vi "GameToIAStateKeeper.vi"(8 "error in (no error)":errorcluster, 11 "Game in":refnum<class "Game.lvclass">) -> (0 "error out":errorcluster, 2 "IA State out":T1={"our_robots"=[], "enemy_robots"=[], "balls"=[], "geometry"={"line_width"=0, "field_length"=0, "field_width"=0, "boundary_width"=0, "referee_width"=0, "goal_width"=0, "goal_depth"=0, "goal_wall_width"=0, "center_circle_radius"=0, "defense_radius"=0, "defense_stretch"=0, "free_kick_from_defense_dist"=0, "penalty_spot_from_field_line_dist"=0, "penalty_line_from_spot_dist"=0}, "IA Judge"={"stage"="", "command"="", "our_goalie_id"=0.0, "enemy_goalie_id"=0.0, "command enum"=enum."Halt", "Time"=enum."Azul", "Point"={"x"=0.0, "y"=0.0}}, "Received Timestamp"=timestamp(0 s since 1904-01-01), "Events"={"Touch"=FALSE, "Ball out"=FALSE, "id touch"=0.0, "Ball out of \nVision"=FALSE, "Ball inside \nGoalie area"=FALSE, "Robot not responding"=FALSE, "Robots responding status"=[1.0, 1.0, 1.0, 1.0, 1.0, 1.0], "Enemy Ball \nPossession"=FALSE, "Pass State"=FALSE, "id end of pass"=0.0, "Kick"=FALSE, "Id ini Possession"=0.0, "Ball Possesion"=FALSE, "Id Possesion"=0.0, "Direct Kick"=FALSE, "2nd Strk Ativo"=FALSE}}, 3 "Game out":refnum<class "Game.lvclass">, 6 "Parameters.lvclass":refnum<class "Parameters.lvclass">)   [LabVIEW 2023, in "Game.lvclass"]
uses:
  Game.lvclass
  Vision_class/Old vision/SSL Detection Frame Simple Estimator Cameras VelCmd Folder/Core/AI Input.ctl
  Vision_class/Old vision/Controls/AI Robot.ctl
  Vision_class/Old vision/Controls/Functions Enum.ctl
  Controls/estimatives.ctl
  Vision_class/Old vision/Controls/AttackerStates.ctl
  Vision_class/Old vision/Controls/PathDests.ctl
  Vision_class/Old vision/Controls/PathDest.ctl
  Navigation/VSSNavigation/VSSAttackerStates.ctl
  Robot_class/robotKickToStates.ctl
  Robot_class/roles.ctl
  <vilib>/Analysis/Matrix/Datatypes/RealMatrix.ctl
  Navigation/driveMode.ctl
  Vision_class/Old vision/SSL Detection Frame Simple Estimator Cameras VelCmd Folder/Core/AI Ball.ctl
  Vision_class/Old vision/SSL Detection Frame Simple Estimator Cameras VelCmd Folder/Core/Field Size.ctl
  Vision_class/Old vision/SSL Detection Frame Simple Estimator Cameras VelCmd Folder/Core/AI Judge.ctl
  Communication_class/Paths/MessageAI_State Folder/Intel/Command Enum.ctl
  Vision_class/Old vision/SSL Detection Frame Simple Estimator Cameras VelCmd Folder/Util/Events/Events.ctl
  Parameters_class/Parameters.lvclass
  Game.lvclass/Game.ctl
  Team_class/Team.lvclass/Team.ctl
  Object_class/Object.lvclass/Object.ctl
  Ball_class/Ball.lvclass/Ball.ctl
  Events_class/Events.lvclass/Events.ctl
  Referee_class/Referee.lvclass/Referee.ctl
  Robot_class/Robot.lvclass/Robot.ctl
  Robot_class/Read id.vi
  Object_class/Read x.vi
  Object_class/Read y.vi
  Robot_class/Read orientation.vi
  Robot_class/Read est_v_tang.vi
  Robot_class/Read est_v_norm.vi
  Object_class/Read pos_est_x.vi
  Object_class/Read pos_est_y.vi
  Robot_class/Read dribble.vi
  Robot_class/Read path.vi
  Robot_class/Read path_smooth.vi
  Robot_class/Read dest_x.vi
  Robot_class/Read dest_y.vi
  Robot_class/Read dest_orientation.vi
  Robot_class/Read role.vi
  Read Parameters.lvclass.vi
  Read KeeperTeam.vi
  Read EnemyRef.vi
  Read BallRef.vi
  Read EventsRef.vi
  Read FieldRef.vi
  Read Referee.vi
  Read TimeRef.vi
  Referee_class/Read command_from_referee.vi
  Referee_class/Read command_interpreted.vi
  Events_class/Read ball_inside_enemy_goalie_area.vi
  Events_class/Read ball_inside_our_goalie_area.vi
  Events_class/Read ball_out.vi
  Events_class/Read ball_out_of_vision.vi
  Events_class/Read enemy_ball_possesion.vi
  Events_class/Read id_enemy_ball_possesion.vi
  Events_class/Read id_our_balll_possesion.vi
  Events_class/Read id_touch.vi
  Events_class/Read kick.vi
  Events_class/Read our_balll_possesion.vi
  Events_class/Read touch.vi
  Ball_class/Read v_x.vi
  Ball_class/Read v_y.vi
  Team_class/Read RobotRef.vi
  Ball_class/Ball.lvclass
  C:/Users/lucio/Desktop/roboime/SSL_AI/Object_class/Object.lvclass
  Enemy_class/Enemy.lvclass
  C:/Users/lucio/Desktop/roboime/SSL_AI/Team_class/Team.lvclass
  Robot_class/Robot.lvclass
  Ally_class/Ally.lvclass
  Events_class/Events.lvclass
  Field_class/Field.lvclass
  Referee_class/Referee.lvclass
  <vilib>/Analysis/Matrix/NI_Matrix.lvlib
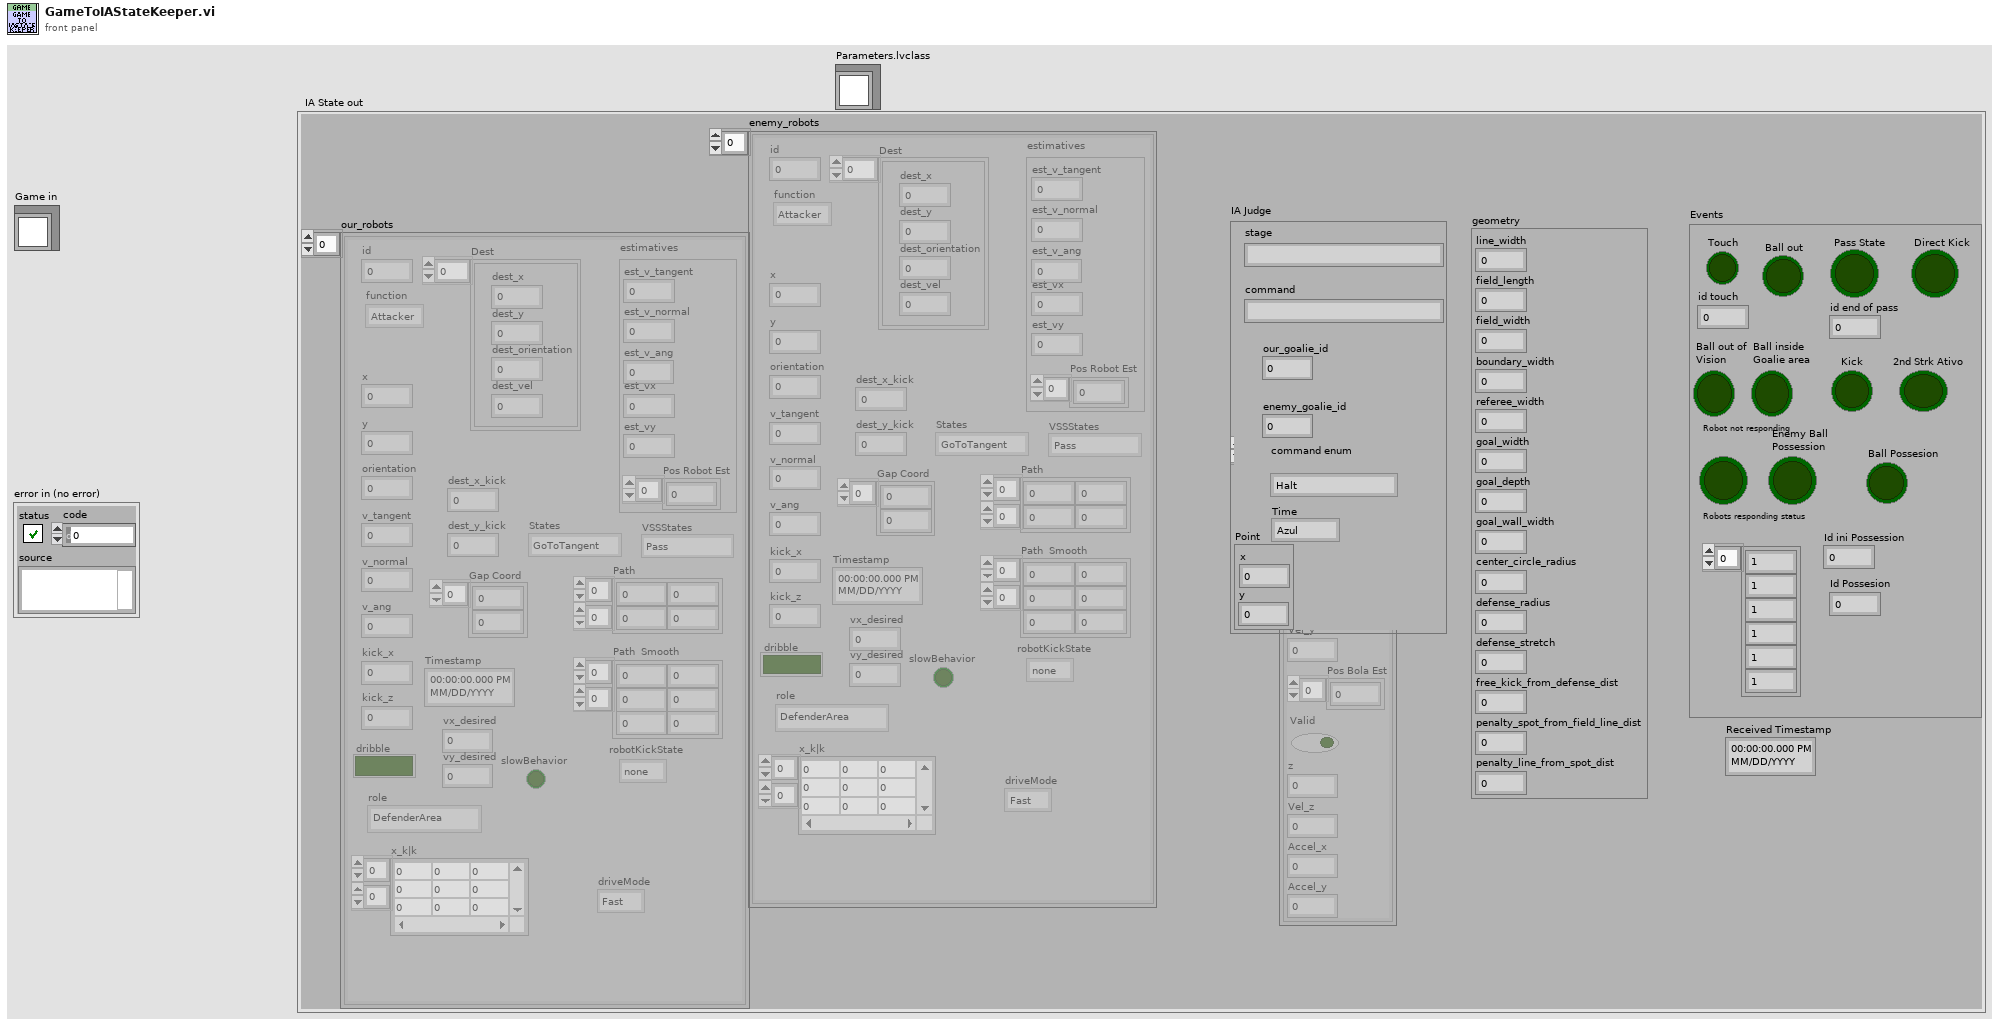
[diagram p1: front panel]
types:
  T1 = typedef "AI Input.ctl" = cluster{"our_robots":T2[], "enemy_robots":T2[], "balls":T13[], "geometry":T14, "IA Judge":T15, "Received Timestamp":timestamp, "Events":T17}
  T2 = typedef "AI Robot.ctl" = cluster{"id":u32, "function":T3, "x":dbl, "y":dbl, "orientation":dbl, "v_tangent":dbl, "v_normal":dbl, "v_ang":dbl, "kick_x":dbl, "kick_z":dbl, "dribble":bool, "Timestamp":timestamp, "estimatives":T4, "dest_x_kick":dbl, "dest_y_kick":dbl, "Gap Coord":dbl[], "States":T5, "Path ":dbl[][], "Path  Smooth":dbl[][], "Dest":T6, "vx_desired":dbl, "vy_desired":dbl, "slowBehavior":bool, "VSSStates":T8, "robotKickState":T9, "role":T10, "x_k|k":T11, "driveMode":T12}
  T3 = typedef "Functions Enum.ctl" = enum16{"2nd Striker", "Attacker", "Goalie", "Defender", "Striker", "Goto 0", "Dummy", "Kicker", "ZigZag 0", "ZigZag 1", "ZigZag 2", "ZigZag 3", "ZigZag 4", "ZigZag 5", "ZigZag 6", "ZigZag 7", "ZigZag 8", ""}
  T4 = typedef "estimatives.ctl" = cluster{"est_v_tangent":dbl, "est_v_normal":dbl, "est_vx":dbl, "est_vy":dbl, "Pos Robot Est":dbl[], "est_v_ang":dbl}
  T5 = typedef "AttackerStates.ctl" = enum16{"Pass", "GoToTangent", "BallGetting", "GoToKick", ""}
  T6 = typedef "PathDests.ctl" = T7[]
  T7 = typedef "PathDest.ctl" = cluster{"dest_x":dbl, "dest_y":dbl, "dest_orientation":dbl, "dest_vel":dbl}
  T8 = typedef "VSSAttackerStates.ctl" = enum16{"Pass", "GoToTangent", "BallGetting", "GoToKick", "Rotate anti-clockwise", "Rotate Clockwise", ""}
  T9 = typedef "robotKickToStates.ctl" = enum16{"shootFromDirect", "avoidCollideBall", "goToBackBall", "none", "walk", "turn", "turnAntiClockWise", "turnClockwise", "oldKickToShoot", "oldKickToGoToBackBall", "shoot"}
  T10 = typedef "roles.ctl" = enum16{"SimpleBallPlacement", "BallPlacementAllyPasser", "BallPlacementAllyReceiver", "BallPlacementEnemy", "5Robots5th", "PassBestReceiver", "5Robots4th", "5Robots3rd", "5Robots2nd", "5Robots1st", "PassBestRobot", "WaitPass", "ABCThirdKicker", "ABCFirstKicker", "ABCSecondKicker", "Tabler", "TableFinalizer", "PrepareRollToPassRoller", "PrepareRollToPassReceiver", "SimplePassRoll", "SimplePassRollReceiver", "PenaltyDefense", "PreparePassReceiver 2", "PreparePassReceiver 1", "PassObserver", "Timeout", "Goto", "ZigZag", "None", "BallOutOfField", "DefenderArea", "Duelist", "AttackerStop", "FollowAttacker", "KeeperRole", "KickPenalty", "AttackerAimGoal", "AttackerBlock", "Marker", "Halt", "Shoot", "PassKicker", "PassReceiver", "TestRole", "PenaltyAttacker"}
  T11 = typedef "NI_Matrix.lvlib/RealMatrix.ctl" = dbl[][]
  T12 = typedef "driveMode.ctl" = enum16{"Fast", "SafeDrive"}
  T13 = typedef "AI Ball.ctl" = cluster{"x":dbl, "y":dbl, "timestamp":timestamp, "Vel_x":dbl, "Vel_y":dbl, "Pos Bola Est":dbl[], "Valid":bool, "z":dbl, "Vel_z":dbl, "Accel_x":dbl, "Accel_y":dbl}
  T14 = typedef "Field Size.ctl" = cluster{"line_width":u32, "field_length":u32, "field_width":u32, "boundary_width":u32, "referee_width":u32, "goal_width":u32, "goal_depth":u32, "goal_wall_width":u32, "center_circle_radius":u32, "defense_radius":u32, "defense_stretch":u32, "free_kick_from_defense_dist":u32, "penalty_spot_from_field_line_dist":u32, "penalty_line_from_spot_dist":u32}
  T15 = typedef "AI Judge.ctl" = cluster{"stage":string, "command":string, "our_goalie_id":dbl, "enemy_goalie_id":dbl, "command enum":T16, "Time":enum16{"Azul", "Amarelo"}, "Point":cluster{"x":sgl, "y":sgl}}
  T16 = typedef "Command Enum.ctl" = enum16{"Halt", "Stop", "Force Start", "PKA Normal Start", "Prepare Kickoff Ally", "PKE Normal Start", "Prepare Kickoff Enemy", "Prepare Penalty Ally", "PPA Normal Start", "Prepare Penalty Enemy", "PPE Normal Start", "Direct Free Enemy", "Direct Free Ally", "Indirect Free Enemy", "Indirect Free Ally", "Timeout Enemy", "Timeout Ally", "Goal Enemy", "Goal Ally", "Ball Placement Enemy", "Ball Placement Ally", "Normal Half Time", "Extra Time Break", "Extra Half Time", "None", "Post Game"}
  T17 = typedef "Events.ctl" = cluster{"Touch":bool, "Ball out":bool, "id touch":dbl, "Ball out of \nVision":bool, "Ball inside \nGoalie area":bool, "Robot not responding":bool, "Robots responding status":dbl[], "Enemy Ball \nPossession":bool, "Pass State":bool, "id end of pass":dbl, "Kick":bool, "Id ini Possession":dbl, "Ball Possesion":bool, "Id Possesion":dbl, "Direct Kick":bool, "2nd Strk Ativo":bool}
  T18 = typedef "command_interpreted.ctl" = enum16{"Goal Ally", "Goal Enemy", "Ball Placement Enemy", "Ball Placement Ally", "Normal Half Time", "Extra Time  Break", "Extra Half Time", "None", "Post Game", "PKA Normal Start", "Prepare Kickoff Ally", "PKE Normal Start", "Prepare Kickoff Enemy", "Force Start", "Halt", "Timeout", "Prepare Penalty Ally", "Prepare Penalty Enemy", "PPA NormalStart", "PPE Normal Start", "Indirect Free Ally", "Direct Free Enemy", "Direct Free Ally", "Indirect Free Enemy", "Stop"}
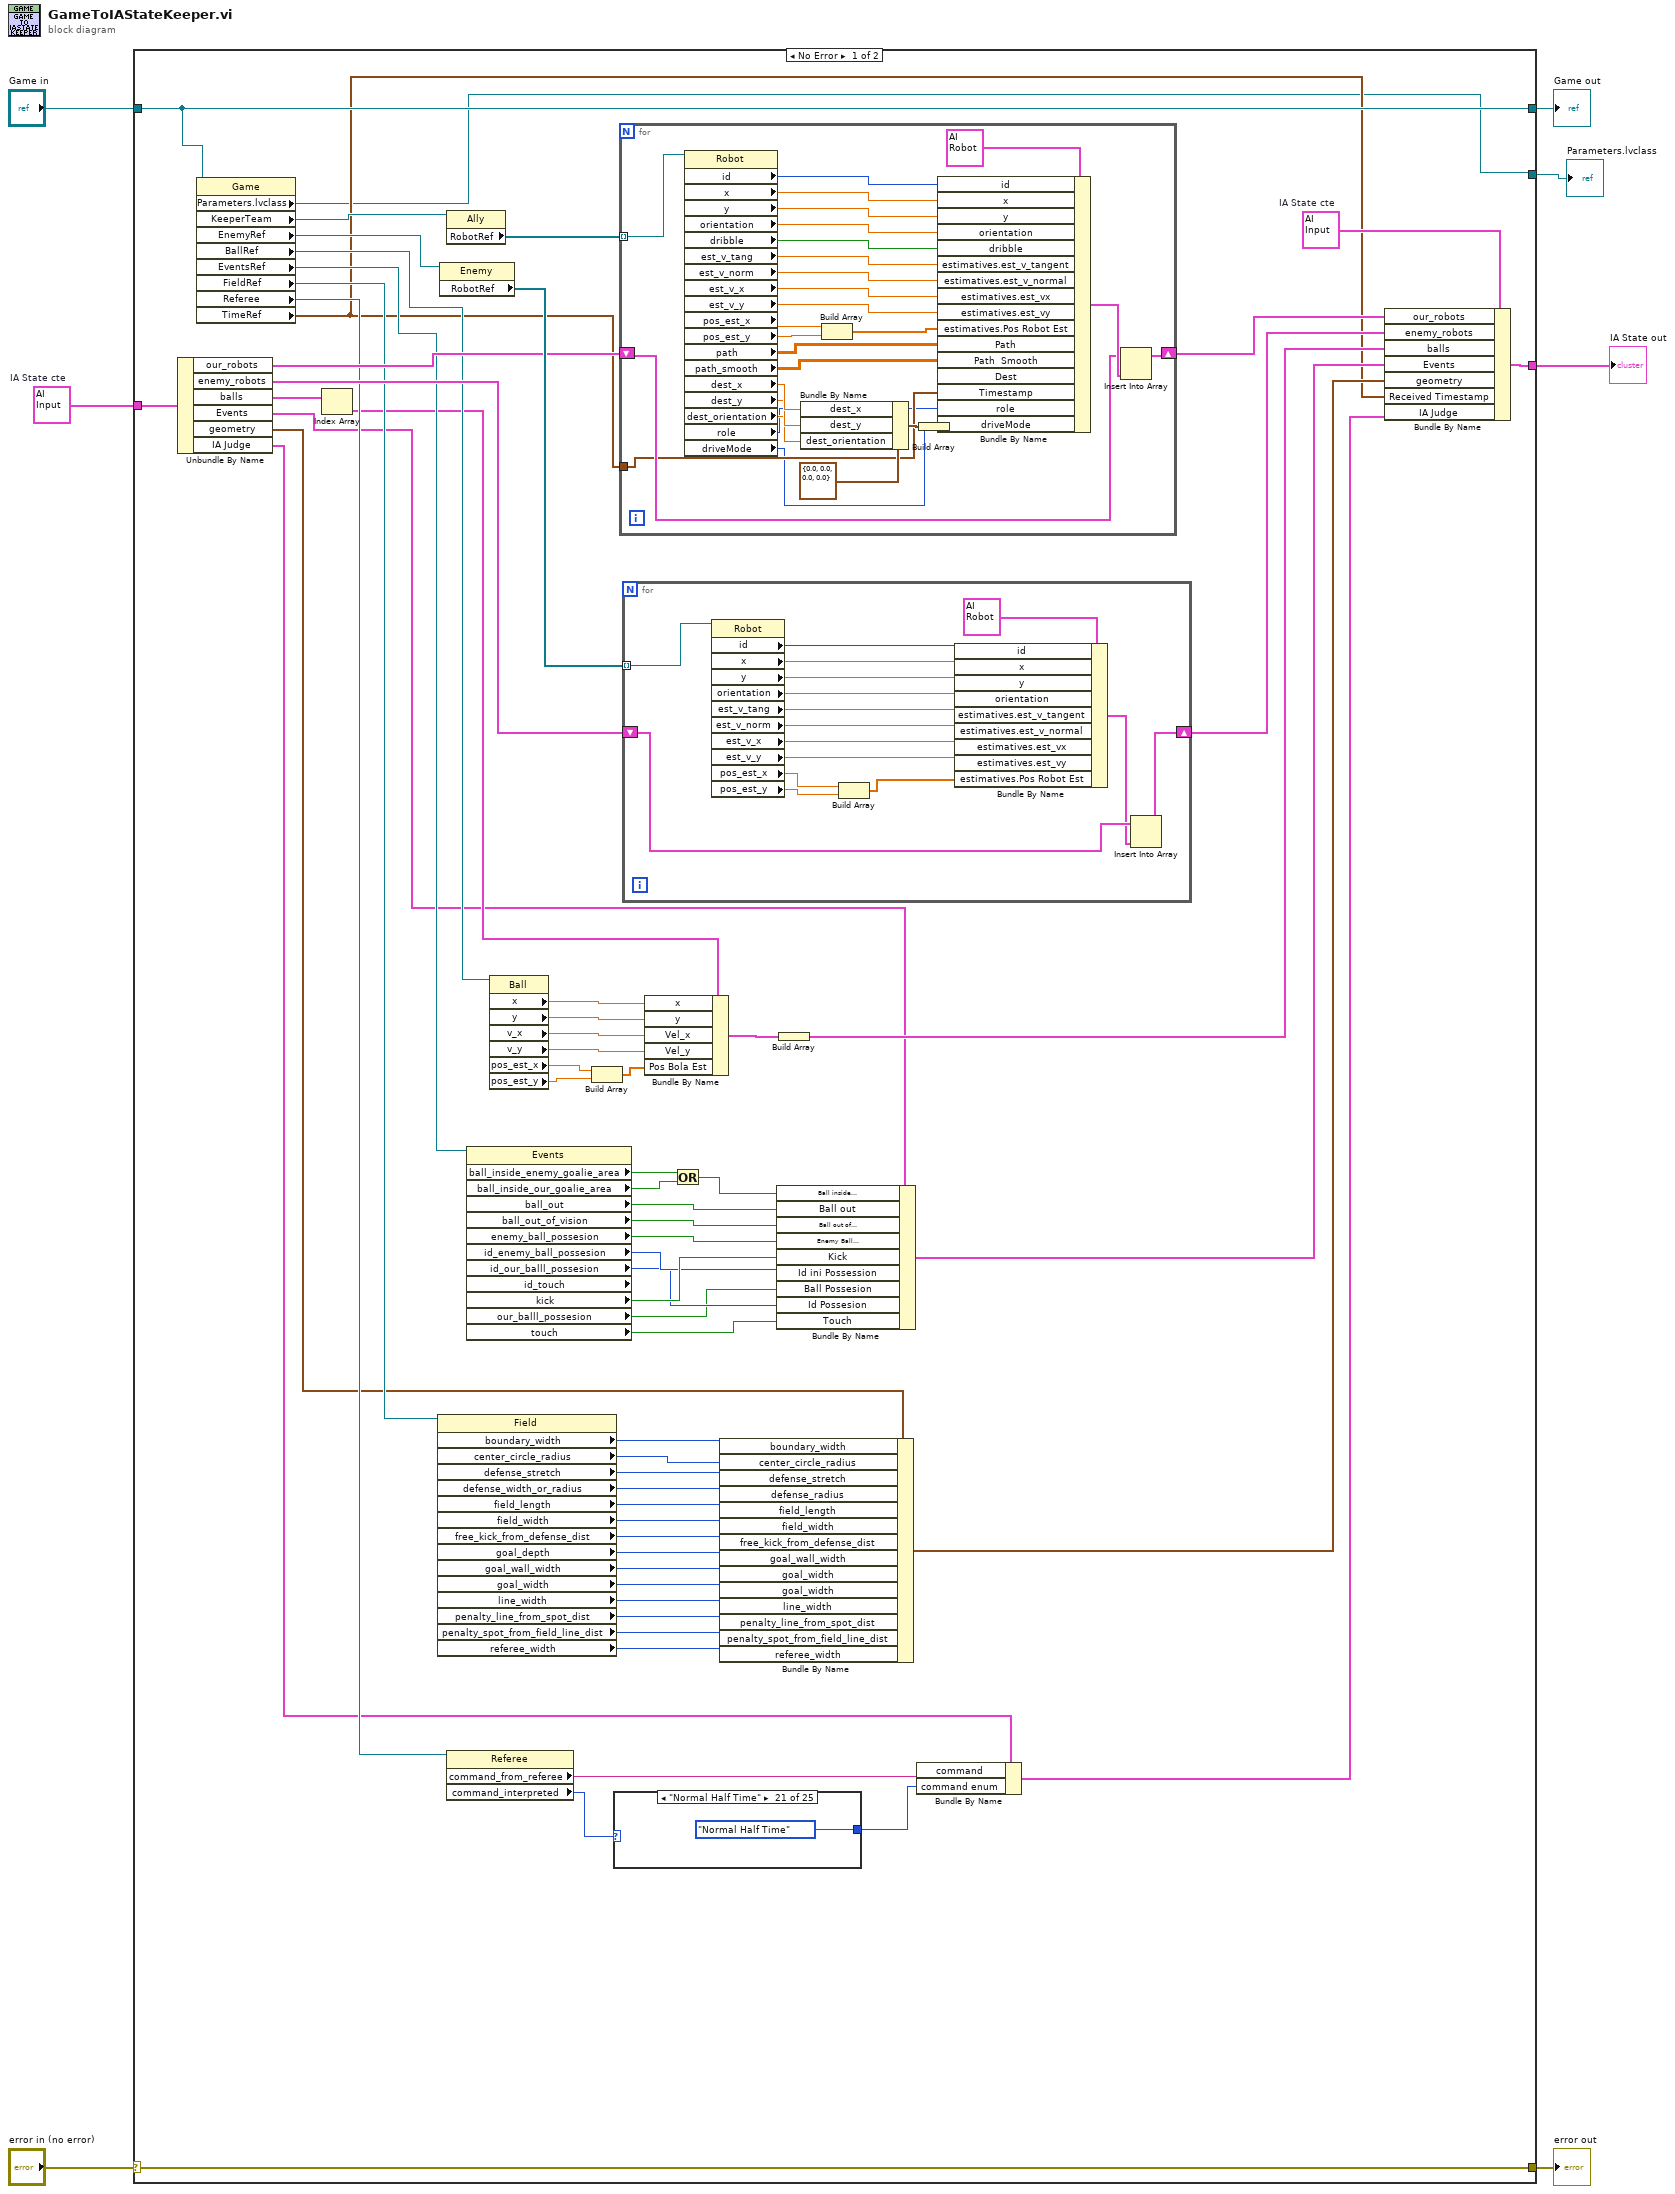
[diagram p0: block diagram]
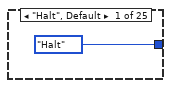
[diagram p2: hidden frame]
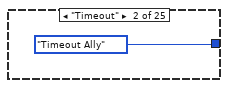
[diagram p3: hidden frame]
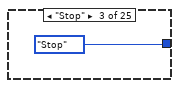
[diagram p4: hidden frame]
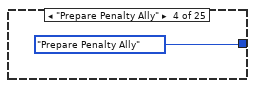
[diagram p5: hidden frame]
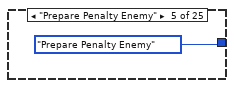
[diagram p6: hidden frame]
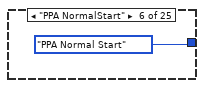
[diagram p7: hidden frame]
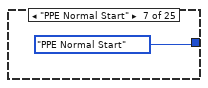
[diagram p8: hidden frame]
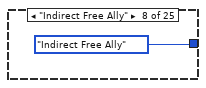
[diagram p9: hidden frame]
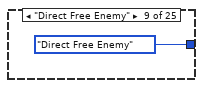
[diagram p10: hidden frame]
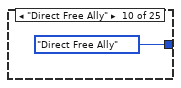
[diagram p11: hidden frame]
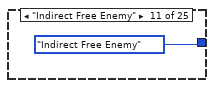
[diagram p12: hidden frame]
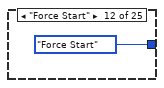
[diagram p13: hidden frame]
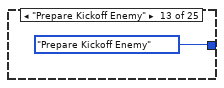
[diagram p14: hidden frame]
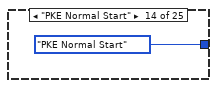
[diagram p15: hidden frame]
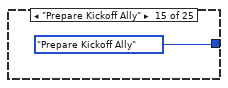
[diagram p16: hidden frame]
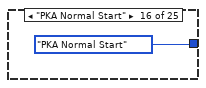
[diagram p17: hidden frame]
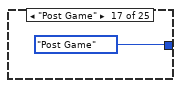
[diagram p18: hidden frame]
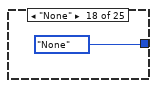
[diagram p19: hidden frame]
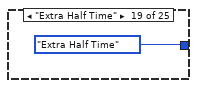
[diagram p20: hidden frame]
diagram:
  w3 = T1 {"our_robots"=[], "enemy_robots"=[], "balls"=[], "geometry"={"line_width"=0, "field_length"=0, "field_width"=0, "boundary_width"=0, "referee_width"=0, "goal_width"=0, "goal_depth"=0, "goal_wall_width"=0, "center_circle_radius"=0, "defense_radius"=0, "defense_stretch"=0, "free_kick_from_defense_dist"=0, "penalty_spot_from_field_line_dist"=0, "penalty_line_from_spot_dist"=0}, "IA Judge"={"stage"="", "command"="", "our_goalie_id"=0.0, "enemy_goalie_id"=0.0, "command enum"=enum."Halt", "Time"=enum."Azul", "Point"={"x"=0.0, "y"=0.0}}, "Received Timestamp"=timestamp(0 s since 1904-01-01), "Events"={"Touch"=FALSE, "Ball out"=FALSE, "id touch"=0.0, "Ball out of \nVision"=FALSE, "Ball inside \nGoalie area"=FALSE, "Robot not responding"=FALSE, "Robots responding status"=[], "Enemy Ball \nPossession"=FALSE, "Pass State"=FALSE, "id end of pass"=0.0, "Kick"=FALSE, "Id ini Possession"=0.0, "Ball Possesion"=FALSE, "Id Possesion"=0.0, "Direct Kick"=FALSE, "2nd Strk Ativo"=FALSE}}  # IA State cte
  n1 = case shown="No Error" "error in (no error)" {
    selector: "error in (no error)" -> [w71 w143]
    tunnel: [w71 w143] -> w6
    tunnel: [w70 w142] -> w4
    tunnel: "Game in" -> [w70 w142]
    tunnel: w3 -> [w65 w141]
    tunnel: [w10 w141] -> w2
    tunnel: [w8 _] -> w1
    frame No Error {
      w61 = T1 {"our_robots"=[], "enemy_robots"=[], "balls"=[], "geometry"={"line_width"=0, "field_length"=0, "field_width"=0, "boundary_width"=0, "referee_width"=0, "goal_width"=0, "goal_depth"=0, "goal_wall_width"=0, "center_circle_radius"=0, "defense_radius"=0, "defense_stretch"=0, "free_kick_from_defense_dist"=0, "penalty_spot_from_field_line_dist"=0, "penalty_line_from_spot_dist"=0}, "IA Judge"={"stage"="", "command"="", "our_goalie_id"=0.0, "enemy_goalie_id"=0.0, "command enum"=enum."Halt", "Time"=enum."Azul", "Point"={"x"=0.0, "y"=0.0}}, "Received Timestamp"=timestamp(0 s since 1904-01-01), "Events"={"Touch"=FALSE, "Ball out"=FALSE, "id touch"=0.0, "Ball out of \nVision"=FALSE, "Ball inside \nGoalie area"=FALSE, "Robot not responding"=FALSE, "Robots responding status"=[], "Enemy Ball \nPossession"=FALSE, "Pass State"=FALSE, "id end of pass"=0.0, "Kick"=FALSE, "Id ini Possession"=0.0, "Ball Possesion"=FALSE, "Id Possesion"=0.0, "Direct Kick"=FALSE, "2nd Strk Ativo"=FALSE}}  # IA State cte
      n2 = Unbundle By Name(w65) -> ("our_robots"=w64:T2[], "enemy_robots"=w63:T2[], "balls"=w18:T13[], "Events"=w16:T17, "geometry"=w15:T14, "IA Judge"=w14:T15)
      n3 = property class="Game"(reference=w70) -> ("Parameters.lvclass"=w8:refnum<class "Parameters.lvclass">, "KeeperTeam"=w69:refnum<class "Ally.lvclass">, "EnemyRef"=w67:refnum<class "Enemy.lvclass">, "BallRef"=w62:refnum<class "Ball.lvclass">, "EventsRef"=w49:refnum<class "Events.lvclass">, "FieldRef"=w36:refnum<class "Field.lvclass">, "Referee"=w20:refnum<class "Referee.lvclass">, "TimeRef"=w9:timestamp)  [unwired: 1 in, 2 out]
      n4 = Index Array(array=w18) -> (element=w17:T13)  [unwired: 1 in]
      n5 = property class="Field"(reference=w36) -> ("boundary_width"=w35:i32, "center_circle_radius"=w34:i32, "defense_stretch"=w33:i32, "defense_width_or_radius"=w32:i32, "field_length"=w31:i32, "field_width"=w30:i32, "free_kick_from_defense_dist"=w29:i32, "goal_depth"=w28:i32, "goal_wall_width"=w27:i32, "goal_width"=w26:i32, "line_width"=w25:i32, "penalty_line_from_spot_dist"=w24:i32, "penalty_spot_from_field_line_dist"=w23:i32, "referee_width"=w22:i32)  [unwired: 1 in, 2 out]
      n6 = property class="Enemy"(reference=w67) -> ("RobotRef"=w66:refnum<class "Robot.lvclass">[])  [unwired: 1 in, 2 out]
      n7 = property class="Ally"(reference=w69) -> ("RobotRef"=w68:refnum<class "Robot.lvclass">[])  [unwired: 1 in, 2 out]
      n8 = property class="Referee"(reference=w20) -> ("command_from_referee"=w19:string, "command_interpreted"=w13:T18)  [unwired: 1 in, 2 out]
      n9 = property class="Events" props=["ball_inside_enemy_goalie_area", "ball_inside_our_goalie_area", "ball_out", "ball_out_of_vision", "enemy_ball_possesion", "id_enemy_ball_possesion", "id_our_balll_possesion", "id_touch", "kick", "our_balll_possesion", "touch"](reference=w49) -> ("ball_inside_enemy_goalie_area"=w47:bool, "ball_inside_our_goalie_area"=w48:bool, "ball_out"=w45:bool, "ball_out_of_vision"=w44:bool, "enemy_ball_possesion"=w43:bool, "id_enemy_ball_possesion"=w41:i32, "id_our_balll_possesion"=w40:i32, "kick"=w42:bool, "our_balll_possesion"=w39:bool, "touch"=w38:bool)  [unwired: 1 in, 3 out]
      n10 = property class="Ball"(reference=w62) -> ("x"=w58:dbl, "y"=w57:dbl, "v_x"=w56:dbl, "v_y"=w55:dbl, "pos_est_x"=w54:dbl, "pos_est_y"=w53:dbl)  [unwired: 1 in, 2 out]
      n11 = Build Array(w54, w53) -> (w52:dbl[])
      n12 = case shown="\"Normal Half Time\"" w13 {
        tunnel: [Command_Enum."Halt" ("command enum") Command_Enum."Timeout Ally" ("command enum") Command_Enum."Stop" ("command enum") Command_Enum."Prepare Penalty Ally" ("command enum") Command_Enum."Prepare Penalty Enemy" ("command enum") Command_Enum."PPA Normal Start" ("command enum") Command_Enum."PPE Normal Start" ("command enum") Command_Enum."Indirect Free Ally" ("command enum") Command_Enum."Direct Free Enemy" ("command enum") Command_Enum."Direct Free Ally" ("command enum") Command_Enum."Indirect Free Enemy" ("command enum") Command_Enum."Force Start" ("command enum") Command_Enum."Prepare Kickoff Enemy" ("command enum") Command_Enum."PKE Normal Start" ("command enum") Command_Enum."Prepare Kickoff Ally" ("command enum") Command_Enum."PKA Normal Start" ("command enum") Command_Enum."Post Game" ("command enum") Command_Enum."None" ("command enum") Command_Enum."Extra Half Time" ("command enum") Command_Enum."Extra Time Break" ("command enum") Command_Enum."Normal Half Time" ("command enum") Command_Enum."Ball Placement Ally" ("command enum") Command_Enum."Ball Placement Enemy" ("command enum") Command_Enum."Goal Enemy" ("command enum") Command_Enum."Goal Ally" ("command enum")] -> w12
        frame "Halt", Default {
        }
        frame "Timeout" {
        }
        frame "Stop" {
        }
        frame "Prepare Penalty Ally" {
        }
        frame "Prepare Penalty Enemy" {
        }
        frame "PPA NormalStart" {
        }
        frame "PPE Normal Start" {
        }
        frame "Indirect Free Ally" {
        }
        frame "Direct Free Enemy" {
        }
        frame "Direct Free Ally" {
        }
        frame "Indirect Free Enemy" {
        }
        frame "Force Start" {
        }
        frame "Prepare Kickoff Enemy" {
        }
        frame "PKE Normal Start" {
        }
        frame "Prepare Kickoff Ally" {
        }
        frame "PKA Normal Start" {
        }
        frame "Post Game" {
        }
        frame "None" {
        }
        frame "Extra Half Time" {
        }
        frame "Extra Time  Break" {
        }
        frame "Normal Half Time" {
        }
        frame "Ball Placement Ally" {
        }
        frame "Ball Placement Enemy" {
        }
        frame "Goal Enemy" {
        }
        frame "Goal Ally" {
        }
      }
      n13 = for {
        tunnel: w68 -> [w120] mode=indexing
        shift-right: [w121] -> w60
        shift-left: w64 -> [w122]
        tunnel: w9 -> [w99]
        n14 = property class="Robot"(reference=w120) -> ("id"=w119:i32, "x"=w118:dbl, "y"=w117:dbl, "orientation"=w116:dbl, "dribble"=w115:bool, "est_v_tang"=w114:dbl, "est_v_norm"=w113:dbl, "est_v_x"=w112:dbl, "est_v_y"=w111:dbl, "pos_est_x"=w110:dbl, "pos_est_y"=w109:dbl, "path"=w107:dbl[][], "path_smooth"=w106:dbl[][], "dest_x"=w105:dbl, "dest_y"=w104:dbl, "dest_orientation"=w103:dbl, "role"=w98:T10, "driveMode"=w97:T12)  [unwired: 1 in, 2 out]
        n15 = Bundle By Name(cluster=T7 {"dest_x"=0.0, "dest_y"=0.0, "dest_orientation"=0.0, "dest_vel"=0.0} ("element"), "dest_x"=w105, "dest_y"=w104, "dest_orientation"=w103) -> (w101:T7)
        n16 = Build Array(w110, w109) -> (w108:dbl[])
        n17 = Build Array(w101) -> (w100:T7[])
        n18 = Bundle By Name(cluster=T2 {"id"=0, "function"=enum."Attacker", "x"=0.0, "y"=0.0, "orientation"=0.0, "v_tangent"=0.0, "v_normal"=0.0, "v_ang"=0.0, "kick_x"=0.0, "kick_z"=0.0, "dribble"=FALSE, "Timestamp"=timestamp(0 s since 1904-01-01), "estimatives"={"est_v_tangent"=0.0, "est_v_normal"=0.0, "est_vx"=0.0, "est_vy"=0.0, "Pos Robot Est"=[], "est_v_ang"=0.0}, "dest_x_kick"=0.0, "dest_y_kick"=0.0, "Gap Coord"=[], "States"=enum."GoToTangent", "Path "=[], "Path  Smooth"=[], "Dest"=[], "vx_desired"=0.0, "vy_desired"=0.0, "slowBehavior"=FALSE, "VSSStates"=enum."Pass", "robotKickState"=enum."none", "role"=enum."DefenderArea", "x_k|k"=[], "driveMode"=enum."Fast"} ("Robot"), "id"=w119, "x"=w118, "y"=w117, "orientation"=w116, "dribble"=w115, "estimatives.est_v_tangent"=w114, "estimatives.est_v_normal"=w113, "estimatives.est_vx"=w112, "estimatives.est_vy"=w111, "estimatives.Pos Robot Est"=w108, "Path"=w107, "Path  Smooth"=w106, "Dest"=w100, "Timestamp"=w99, "role"=w98, "driveMode"=w97) -> (w123:T2)
        n19 = Insert Into Array(array=w122, new element=w123) -> (w121:T2[])  [unwired: 1 in]
      }
      n20 = for {
        tunnel: w66 -> [w135] mode=indexing
        shift-right: [w125] -> w59
        shift-left: w63 -> [w134]
        n21 = property class="Robot"(reference=w135) -> ("id"=w137:i32, "x"=w138:dbl, "y"=w139:dbl, "orientation"=w140:dbl, "est_v_tang"=w133:dbl, "est_v_norm"=w132:dbl, "est_v_x"=w131:dbl, "est_v_y"=w130:dbl, "pos_est_x"=w129:dbl, "pos_est_y"=w128:dbl)  [unwired: 1 in, 2 out]
        n22 = Build Array(w129, w128) -> (w127:dbl[])
        n23 = Bundle By Name(cluster=T2 {"id"=0, "function"=enum."Attacker", "x"=0.0, "y"=0.0, "orientation"=0.0, "v_tangent"=0.0, "v_normal"=0.0, "v_ang"=0.0, "kick_x"=0.0, "kick_z"=0.0, "dribble"=FALSE, "Timestamp"=timestamp(0 s since 1904-01-01), "estimatives"={"est_v_tangent"=0.0, "est_v_normal"=0.0, "est_vx"=0.0, "est_vy"=0.0, "Pos Robot Est"=[], "est_v_ang"=0.0}, "dest_x_kick"=0.0, "dest_y_kick"=0.0, "Gap Coord"=[], "States"=enum."GoToTangent", "Path "=[], "Path  Smooth"=[], "Dest"=[], "vx_desired"=0.0, "vy_desired"=0.0, "slowBehavior"=FALSE, "VSSStates"=enum."Pass", "robotKickState"=enum."none", "role"=enum."DefenderArea", "x_k|k"=[], "driveMode"=enum."Fast"} ("Robot"), "id"=w137, "x"=w138, "y"=w139, "orientation"=w140, "estimatives.est_v_tangent"=w133, "estimatives.est_v_normal"=w132, "estimatives.est_vx"=w131, "estimatives.est_vy"=w130, "estimatives.Pos Robot Est"=w127) -> (w126:T2)
        n24 = Insert Into Array(array=w134, new element=w126) -> (w125:T2[])  [unwired: 1 in]
      }
      n25 = Bundle By Name(cluster=w17, "x"=w58, "y"=w57, "Vel_x"=w56, "Vel_y"=w55, "Pos Bola Est"=w52) -> (w51:T13)
      n26 = Or(x=w47, y=w48) -> (x .or. y?=w46:bool)
      n27 = Bundle By Name(cluster=w15, "boundary_width"=w35, "center_circle_radius"=w34, "defense_stretch"=w33, "defense_radius"=w32, "field_length"=w31, "field_width"=w30, "free_kick_from_defense_dist"=w29, "goal_wall_width"=w28, "goal_width"=w27, "goal_width"=w26, "line_width"=w25, "penalty_line_from_spot_dist"=w24, "penalty_spot_from_field_line_dist"=w23, "referee_width"=w22) -> (w21:T14)
      n28 = Bundle By Name(cluster=w16, "Ball inside \nGoalie area"=w46, "Ball out"=w45, "Ball out of \nVision"=w44, "Enemy Ball \nPossession"=w43, "Kick"=w42, "Id ini Possession"=w41, "Ball Possesion"=w39, "Id Possesion"=w40, "Touch"=w38) -> (w37:T17)
      n29 = Build Array(w51) -> (w50:T13[])
      n30 = Bundle By Name(cluster=w14, "command"=w19, "command enum"=w12) -> (w11:T15)
      n31 = Bundle By Name(cluster=w61, "our_robots"=w60, "enemy_robots"=w59, "balls"=w50, "Events"=w37, "geometry"=w21, "Received Timestamp"=w9, "IA Judge"=w11) -> (w10:T1)
    }
    frame Error {
    }
  }
  "error out" <- w6
  "Game out" <- w4
  "IA State out" <- w2
  "Parameters.lvclass" <- w1
